vi "Tektronix AFG 1000 Series Waveform Burst.vi"() -> ()   [LabVIEW 2016]
doc: "Demonstrates how to configure burst mode and trigger source.\n\nNote:\n\nFor external trigger source an external trigger input would be required."
uses:
  <instrlib>/Tektronix AFG 1000 Series/Tektronix AFG 1000 Series.lvlib
panel:
  in  "Channel (1: Channel 1)":u16(ring)=1 items=["Channel 1"=1, "Channel2"=2]
  in  "Frequency (1000 Hz)":dbl=1000.0
  in  "DC Offset (0 V)":dbl
  in  "Gain (1 V)":dbl=1.0
  in  "Enable Burst (T: Enable)":bool=TRUE
  in  "Built-in Waveform Name (\"Cardiac\")":string="Cardiac"
  in  "Burst Count (1)":i32=1
  in  "Burst Mode (0: Triggered)":u16(ring) items=["Triggered", "Gated"]
  in  "VISA resource name":refnum<visa-resource-name>
  # "(c) 2016 National Instruments.  ALL RIGHTS RESERVED."
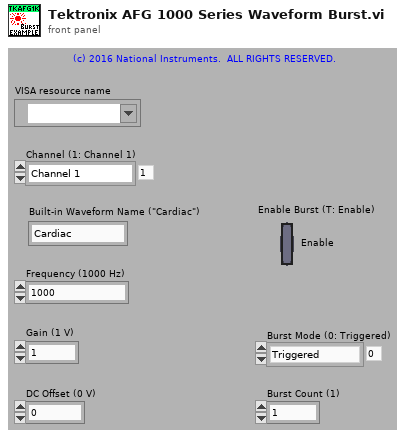
[diagram p1: front panel]
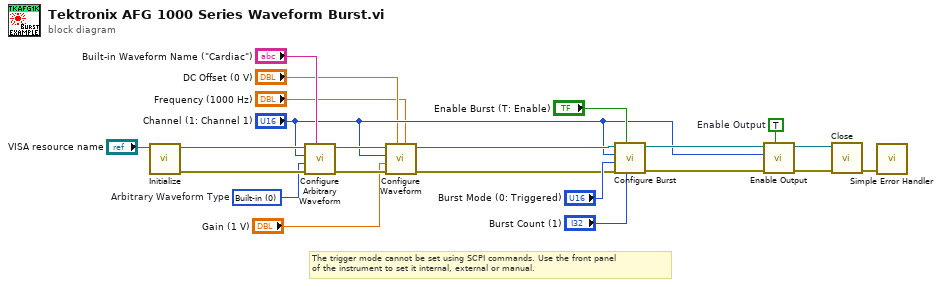
[diagram p0: block diagram]
diagram:
  w4 = u16 0 items=["Built-in", "User Waveform", "Edit Memory", "EFile"]  # Arbitrary Waveform Type
  w20 = TRUE  # Enable Output
  # "The trigger mode cannot be set using SCPI commands. Use the front panel\nof the instrument to set it internal, external or manual."
  n1 = call <instrlib>:"Initialize.vi"("VISA resource name"="VISA resource name") -> ("error out"=w16:errorcluster, "VISA resource name out"=w17:refnum<visa-resource-name>)  [unwired: 9 in]
  n2 = call <instrlib>:"Configure Arbitrary Waveform.vi"("Built-in Waveform Name (\"StairDown\")"="Built-in Waveform Name (\"Cardiac\")", "error in (no error)"=w16, "Arbitrary Waveform Type (0: Built-in)"=w4, "Channel (1: Channel 1)"="Channel (1: Channel 1)", "VISA resource name"=w17) -> ("error out"=w9:errorcluster, "VISA resource name out"=w8:refnum<visa-resource-name>)  [unwired: 5 in]
  n3 = call <instrlib>:"Configure Waveform.vi"("Frequency (1000 Hz)"="Frequency (1000 Hz)", "DC Offset (0.00 V)"="DC Offset (0 V)", "error in (no error)"=w9, "Amplitude (1 Vpp)"="Gain (1 V)", "Channel (1 Channel 1)"="Channel (1: Channel 1)", "VISA resource name"=w8) -> ("error out"=w7:errorcluster, "VISA resource name out"=w6:refnum<visa-resource-name>)  [unwired: 4 in]
  n4 = call <instrlib>:"Configure Burst.vi"("Burst Count (1)"="Burst Count (1)", "Enable Burst (T: Enable)"="Enable Burst (T: Enable)", "error in (no error)"=w7, "Burst Mode (0: Triggered)"="Burst Mode (0: Triggered)", "Channel (1 Channel 1)"="Channel (1: Channel 1)", "VISA resource name"=w6) -> ("error out"=w12:errorcluster, "VISA resource name out"=w13:refnum<visa-resource-name>)  [unwired: 4 in]
  n5 = call <instrlib>:"Enable Output.vi"("Enable Output (T: Enable)"=w20, "error in (no error)"=w12, "Channel (1: Channel 1)"="Channel (1: Channel 1)", "VISA resource name"=w13) -> ("error out"=w14:errorcluster, "VISA resource name out"=w15:refnum<visa-resource-name>)  [unwired: 6 in]
  n6 = call <instrlib>:"Close.vi"("error in (no error)"=w14, "VISA resource name"=w15) -> ("error out"=w22:errorcluster)  [unwired: 9 in]
  n7 = call <vilib>:"Simple Error Handler.vi"("error in (no error)"=w22) -> ()  [unwired: 4 in, 5 out]
